vi "ALTS-2015 Scanner Driver.vi"(7 "Operation":T1, 8 "error in (no error)":errorcluster, 11 "Scanner 2?  (Scanner1)":bool) -> (0 "error out":errorcluster, 3 "Serial No":string)   [LabVIEW 2013]
doc: "Copyright © 2005, Soliton Technologies.\nAll rights reserved."
uses:
  Controls/ALTS-2015 Scanner Driver Options.ctl
  7 Spindle System/Software/Source Code/Controls/7 Spindle - LV2GBL Options.ctl
  <vilib>/Utility/file.llb/Read From Spreadsheet File (string).vi
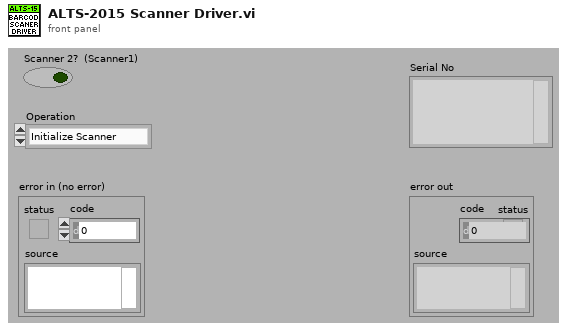
[diagram p1: front panel]
types:
  T1 = typedef "ALTS-2015 Scanner Driver Options.ctl" = enum16{"Initialize Scanner", "Read Scanner", "Close Scanner"}
  T2 = typedef "7 Spindle - LV2GBL Options.ctl" = enum16{"Read all", "Write all"}
  T3 = typedef "ALTS-2015 INI Configuration Cluster.ctl" = cluster{"Station Details":cluster{"Sensor Name 1":string, "Sensor Name 2":string, "Sensor Name 3":string, "Sensor Name 4":string, "Station1 Enable":bool, "Station2 Enable":bool, "Station3 Enable":bool, "Station4 Enable":bool}, "Database":cluster{"Database Connection Link":path, "Result Procedure":string, "User":string, "Password":string, "Prompt":bool, "Station 1 LT Result DB DSN Path":path, "Station 2 LT Result DB DSN Path":path, "Station 3 LT Result DB DSN Path":path, "Station 4 LT Result DB DSN Path":path}, "Simulation":cluster{"Simulate DAQ Hardware":bool, "Simulate Result DB Write":bool, "Scanner Simulation":bool, "Simu. Scanner Path":path, "Simulate OPC":bool, "Simulate LeakTek DB":bool}, "Barcode Scanner1":cluster{"Scanner IP":string, "Scanner Port":u16, "#Bytes to Read":i32}, "Barcode Scanner2":cluster{"Enabled?":bool, "Scanner IP":string, "Scanner Port":u16, "#Bytes to Read":i32}}
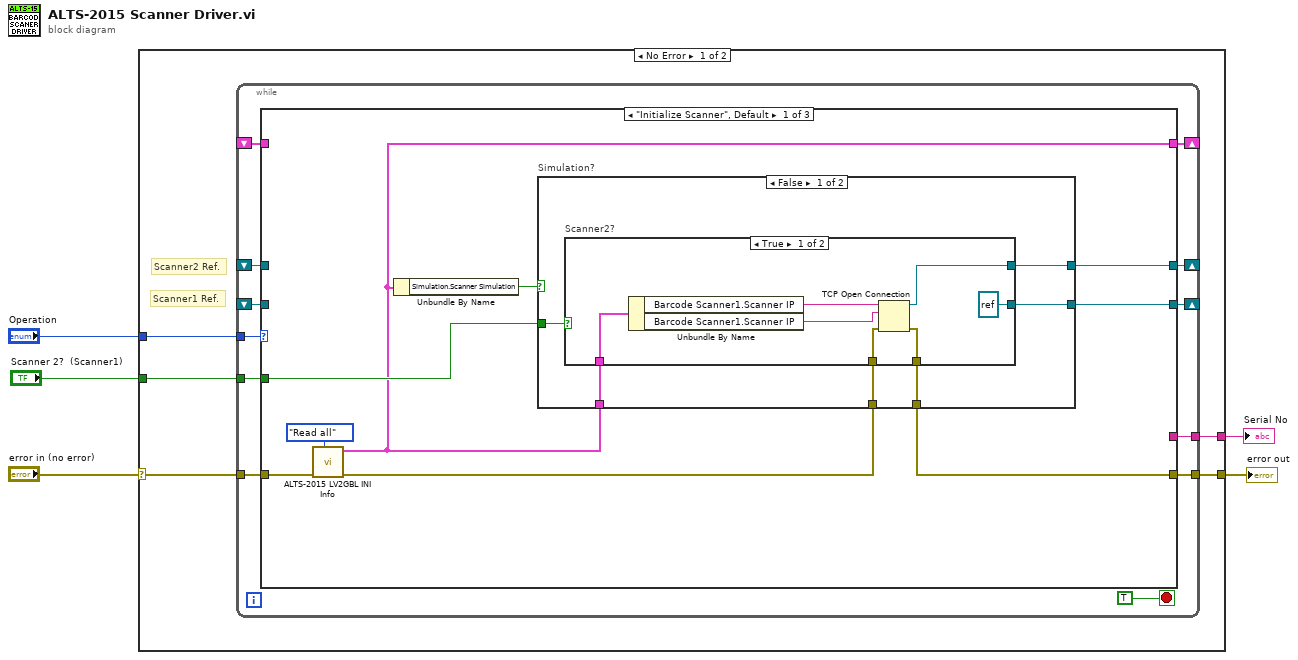
[diagram p0: block diagram]
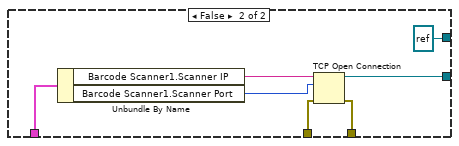
[diagram p2: hidden frame]
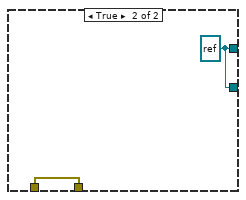
[diagram p3: hidden frame]
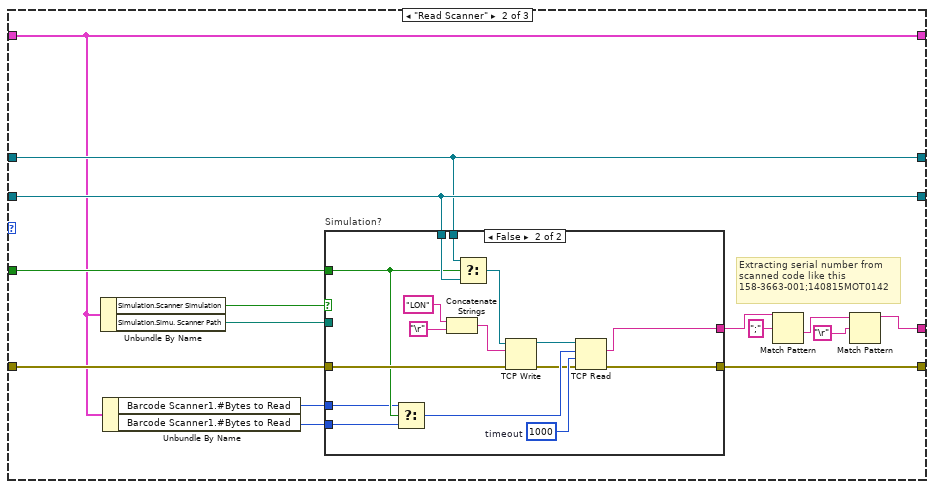
[diagram p4: hidden frame]
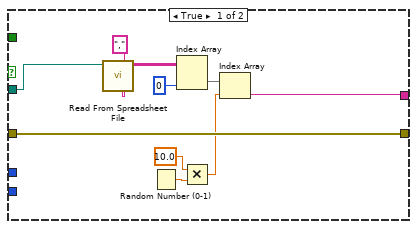
[diagram p5: hidden frame]
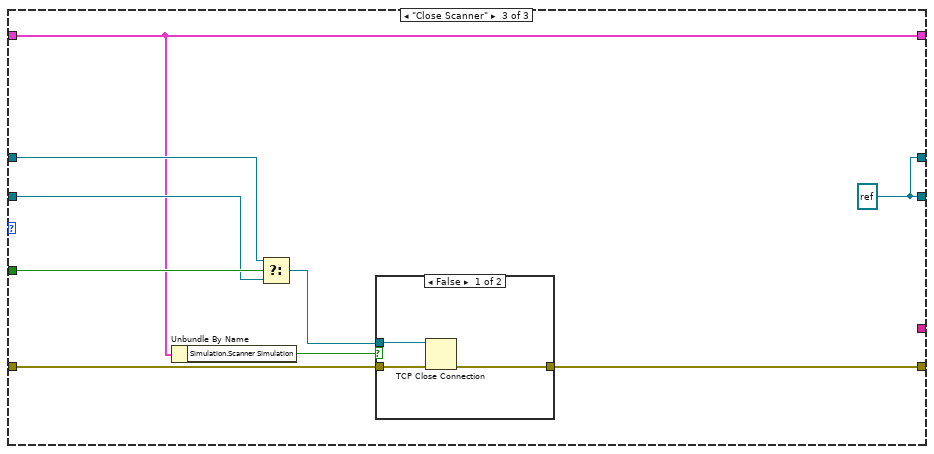
[diagram p6: hidden frame]
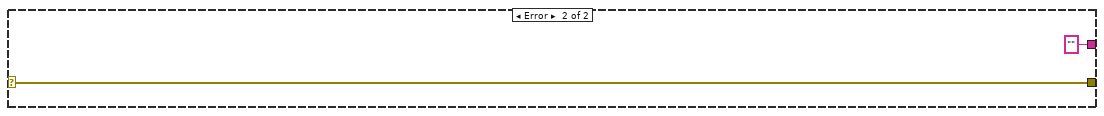
[diagram p8: hidden frame]
diagram:
  n1 = case shown="No Error" "error in (no error)" {
    selector: "error in (no error)" -> [w9 w109]
    tunnel: [w10 w109] -> w4
    tunnel: "Operation" -> [w8 _]
    tunnel: "Scanner 2?  (Scanner1)" -> [w7 _]
    tunnel: [w6 "" ("String")] -> w1
    frame No Error {
      # "Scanner1 Ref."
      # "Scanner2 Ref."
      n2 = while {
        tunnel: [w21] -> w10
        shift-right: [w20] -> _
        shift-left: _ -> [w19]
        tunnel: w9 -> [w18]
        tunnel: w8 -> [w17]
        tunnel: w7 -> [w16]
        shift-right: [w15] -> _
        shift-left: _ -> [w14]
        tunnel: [w13] -> w6
        shift-right: [w12] -> _
        shift-left: _ -> [w11]
        stop <- TRUE stop-if-true
        n3 = case shown="\"Initialize Scanner\", Default" w17 {
          tunnel: w18 -> [w31 w65 w102]
          tunnel: [w27 w68 w103] -> w21
          tunnel: [w29 w66 w96] -> w20
          tunnel: w19 -> [_ w66 w98]
          tunnel: w16 -> [w30 w64 w100]
          tunnel: [w26 w67 w96] -> w15
          tunnel: w14 -> [_ w67 w99]
          tunnel: [_ w55 _] -> w13
          tunnel: [w24 w54 w95] -> w12
          tunnel: w11 -> [_ w54 w95]
          frame "Initialize Scanner", Default {
            n4 = call "ALTS-2015 LV2GBL INI Info.vi"("Options"=7_Spindle_-_LV2GBL_Options."Read all", "error in"=w31) -> ("error out"=w28:errorcluster, "Configuration Cluster Out"=w24:T3)  [unwired: 8 in]
            n5 = Unbundle By Name(w24) -> ("Simulation.Scanner Simulation"=w25:bool)
            n6 = case "Simulation?" shown="False" w25 {
              tunnel: w24 -> [w37 _]
              tunnel: w30 -> [w36 _]
              tunnel: [w35 w53] -> w29
              tunnel: w28 -> [w34 w52]
              tunnel: [w33 w52] -> w27
              tunnel: [w32 w53] -> w26
              frame False {
                n7 = case "Scanner2?" shown="True" w36 {
                  tunnel: w37 -> [w44 w51]
                  tunnel: [w39 refnum<k5> refnum ("connection ID")] -> w35
                  tunnel: w34 -> [w41 w48]
                  tunnel: [w40 w47] -> w33
                  tunnel: [refnum<k5> refnum ("connection ID") w46] -> w32
                  frame True {
                    n8 = Unbundle By Name(w44) -> ("Barcode Scanner1.Scanner IP"=w43:string, "Barcode Scanner1.Scanner IP"=w42:string)
                    n9 = TCP Open Connection(address=w43, remote port or service name=w42, error in (no error)=w41) -> (connection ID=w39:refnum<k5>, error out=w40:errorcluster)  [unwired: 2 in]
                  }
                  frame False {
                    n10 = Unbundle By Name(w51) -> ("Barcode Scanner1.Scanner IP"=w50:string, "Barcode Scanner1.Scanner Port"=w49:u16)
                    n11 = TCP Open Connection(address=w50, remote port or service name=w49, error in (no error)=w48) -> (connection ID=w46:refnum<k5>, error out=w47:errorcluster)  [unwired: 2 in]
                  }
                }
              }
              frame True {
                w53 = refnum<k5> refnum ("connection ID")
              }
            }
          }
          frame "Read Scanner" {
            # "Extracting serial number from \nscanned code like this \n158-3663-001;140815MOT0142"
            n12 = Unbundle By Name(w54) -> ("Simulation.Scanner Simulation"=w61:bool, "Simulation.Simu. Scanner Path"=w60:path)
            n13 = Unbundle By Name(w54) -> ("Barcode Scanner1.#Bytes to Read"=w63:i32, "Barcode Scanner1.#Bytes to Read"=w62:i32)
            n14 = case "Simulation?" shown="False" w61 {
              tunnel: [w78 w89] -> w68
              tunnel: w67 -> [_ w88]
              tunnel: w66 -> [_ w87]
              tunnel: [w69 w79] -> w59
              tunnel: w65 -> [w78 w85]
              tunnel: w64 -> [_ w84]
              tunnel: w63 -> [_ w83]
              tunnel: w62 -> [_ w82]
              tunnel: w60 -> [w70 _]
              frame True {
                n15 = call-poly <vilib>:"Read From Spreadsheet File.vi"("delimiter (\\t)"="," ("delimiter (\\t)"), "file path (dialog if empty)"=w70) -> ("all rows"=w73:string[][])  [unwired: 5 in, 4 out]
                n16 = Random Number (0-1)() -> (number: 0 to 1=w75:dbl)
                n17 = Index Array(array=w73, index (col)=0 ("disabled index (col)")) -> (element=w74:string[])  [unwired: 1 in]
                n18 = Multiply(x=10.0, y=w75) -> (x*y=w76:dbl)
                n19 = Index Array(array=w74, index=w76) -> (element=w69:string)
              }
              frame False {
                w94 = 1000  # timeout
                n20 = Select(t=w83, s=w84, f=w82) -> (s? t:f=w81:i32)
                n21 = Concatenate Strings("LON", "\r" ("string")) -> (w92:string)
                n22 = Select(t=w87, s=w84, f=w88) -> (s? t:f=w86:refnum<k5>)
                n23 = TCP Write(connection ID=w86, data in=w92, error in (no error)=w85) -> (connection ID out=w91:refnum<k5>, error out=w80:errorcluster)  [unwired: 2 out]
                n24 = TCP Read(connection ID=w91, bytes to read=w81, error in (no error)=w80, 9:w94) -> (data out=w79:string, error out=w89:errorcluster)  [unwired: 1 in, 1 out]
              }
            }
            n25 = Match Pattern(string=w59, regular expression=";") -> (after substring=w56:string)  [unwired: 1 in, 3 out]
            n26 = Match Pattern(string=w56, regular expression="\r" ("string")) -> (before substring=w55:string)  [unwired: 1 in, 3 out]
          }
          frame "Close Scanner" {
            w96 = refnum<k5> refnum ("connection ID")
            n27 = Unbundle By Name(w95) -> ("Simulation.Scanner Simulation"=w101:bool)
            n28 = Select(t=w98, s=w100, f=w99) -> (s? t:f=w97:refnum<k5>)
            n29 = case shown="False" w101 {
              tunnel: [w105 w107] -> w103
              tunnel: w97 -> [w104 _]
              tunnel: w102 -> [w106 w107]
              frame False {
                n30 = TCP Close Connection(connection ID=w104, error in (no error)=w106) -> (error out=w105:errorcluster)  [unwired: 1 in, 1 out]
              }
              frame True {
              }
            }
          }
        }
      }
    }
    frame Error {
    }
  }
  "error out" <- w4
  "Serial No" <- w1
